vi "4Pi 4Pi Modes - Get Image ROI.vi"(0 "Camera Notifier Name":string, 7 "Image Ref":T1, 11 "Frame Accums.":u16) -> (8 "Image Out":u16[][](array[numeric]))   [LabVIEW 2016]
uses:
  <vilib>/vision/Image Controls.llb/IMAQ Image.ctl
  Display Module/Display Module TypeDefs/ROI Descriptor.ctl
  Device Library/Cameras/Camera Controls/Generic Camera Actions.ctl
  Device Library/Cameras/Camera Controls/Camera IMAQ Key Info.ctl
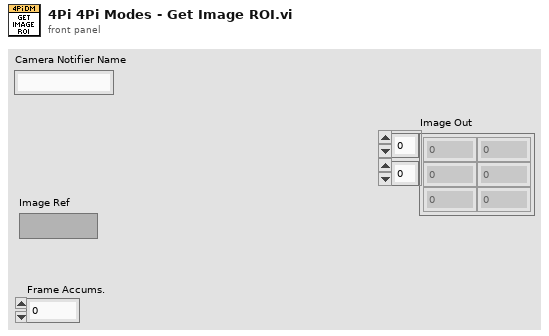
[diagram p1: front panel]
types:
  T1 = typedef "IMAQ Image.ctl" = refnum<image>
  T2 = typedef "Generic Camera Actions.ctl" = enum16{"Status", "Live Preview", "Capture", "Abort", "Set Exposure Time (s)", "Get Exposure Time (s)", "Record Settings", "Set ROI", "Get ROI", "Defect Correction On/Off", "Cooler On/Off", "Fan On/Off", "Quti"}
  T3 = typedef "ROI Descriptor.ctl" = cluster{"Global Rectangle":i32[], "Contours":cluster{"Contour Type":u32, "ROI Type":u32, "Points":i32[]}[]}
  T4 = typedef "Camera IMAQ Key Info.ctl" = cluster{"Frame":u32, "Sensor Height":i32, "Sensor Width":i32, "ROI Height":i32, "ROI Width":i32, "ROI Enable?":bool, "Bit per Pixel":u8}
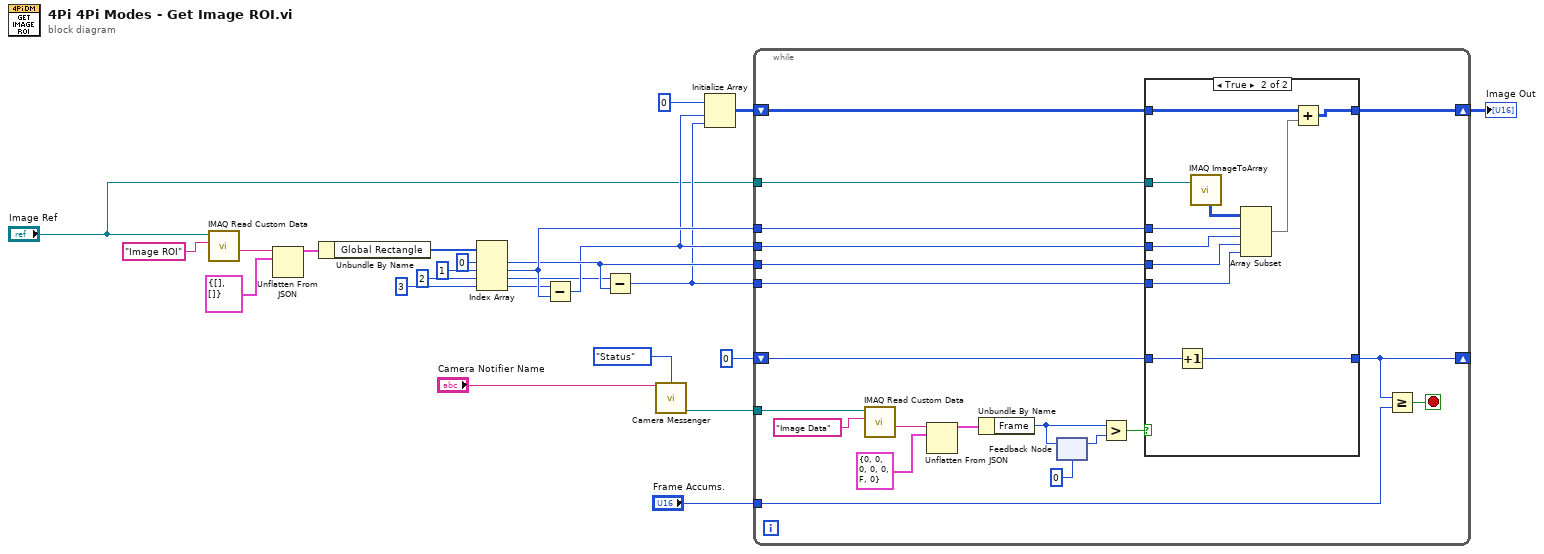
[diagram p0: block diagram]
diagram:
  n1 = call "IMAQ Read Custom Data"("Key"="Image ROI", "Image"="Image Ref") -> ("Custom Data Out"=w13:string)  [unwired: 7 in, 2 out]
  n2 = Unflatten From JSON(JSON string=w13, type and defaults=T3 {"Global Rectangle"=[], "Contours"=[]} ("Image ROI Descriptor")) -> (value=w11:T3)  [unwired: 5 in, 1 out]
  n3 = Unbundle By Name(w11) -> ("Global Rectangle"=w10:i32[])
  n4 = Index Array(array=w10, index #1=0 ("index"), index #2=1 ("index"), index #3=2 ("index"), index #4=3 ("index")) -> (element #1=w18:i32, element #2=w19:i32, element #3=w4:i32, element #4=w5:i32)
  n5 = Subtract(x=w5, y=w19) -> (x-y=w17:i32)
  n6 = Subtract(x=w4, y=w18) -> (x-y=w16:i32)
  n7 = call "Camera Messenger.vi"("Notifier Name"="Camera Notifier Name", "General Camera Actions"=Generic_Camera_Actions."Status") -> ("Image Ref"=w23:T1)  [unwired: 8 in, 5 out]
  n8 = Initialize Array(u16 0, w17, w16) -> (w21:u16[][])
  n9 = while {
    tunnel: w23 -> [w40]
    shift-right: [w34] -> _
    shift-left: u16 0 -> [w35]
    tunnel: "Image Ref" -> [w32]
    shift-right: [w26] -> w15
    shift-left: w21 -> [w27]
    tunnel: w19 -> [w31]
    tunnel: w17 -> [w30]
    tunnel: w18 -> [w29]
    tunnel: w16 -> [w28]
    tunnel: "Frame Accums." -> [w25]
    stop <- w33 stop-if-true
    n10 = call "IMAQ Read Custom Data"("Key"="Image Data", "Image"=w40) -> ("Custom Data Out"=w42:string)  [unwired: 7 in, 2 out]
    n11 = Unflatten From JSON(JSON string=w42, type and defaults=T4 {"Frame"=0, "Sensor Height"=0, "Sensor Width"=0, "ROI Height"=0, "ROI Width"=0, "ROI Enable?"=FALSE, "Bit per Pixel"=0} ("Camera IMAQ Key Info")) -> (value=w44:T4)  [unwired: 5 in, 1 out]
    n12 = Unbundle By Name(w44) -> ("Frame"=w37:u32)
    n13 = feedback #1(u32 0 ("Frame")) -> (w39:u32)
    n14 = feedback-in #1(w37) -> ()
    n15 = Greater?(x=w37, y=w39) -> (0:w36:bool)
    n16 = case shown="True" w36 {
      tunnel: w35 -> [w46 w57]
      tunnel: [w46 w56] -> w34
      tunnel: w32 -> [_ w55]
      tunnel: w31 -> [_ w53]
      tunnel: w30 -> [_ w52]
      tunnel: w29 -> [_ w51]
      tunnel: w28 -> [_ w50]
      tunnel: w27 -> [w45 w49]
      tunnel: [w45 w47] -> w26
      frame False {
      }
      frame True {
        n17 = Increment(x=w57) -> (x+1=w56:u16)
        n18 = call "IMAQ ImageToArray"("Image"=w55) -> ("Image Pixels (U16)"=w54:u16[][])  [unwired: 3 in, 4 out]
        n19 = Array Subset(array=w54, index (row)=w53, length (row)=w52, index (col)=w51, length (col)=w50) -> (w48:u16[][])
        n20 = Add(x=w49, y=w48) -> (x+y=w47:u16[][])
      }
    }
    n21 = Greater Or Equal?(x=w34, y=w25) -> (x >= y?=w33:bool)
  }
  "Image Out" <- w15
